vi "Write_Output.vi"(8 "Error_In":errorcluster, 10 "Output":dbl, 11 "Calculator_In":refnum<class "Calculator.lvclass">) -> (0 "Error_Out":errorcluster, 3 "Calculator_Out":refnum<class "Calculator.lvclass">)   [LabVIEW 2023, in "Calculator.lvclass"]
doc: "Used to write the data of output of calculator class"
uses:
  Calculator.lvclass
  Calculator.lvclass/Calculator.ctl
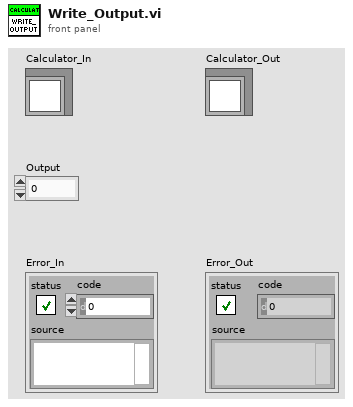
[diagram p1: front panel]
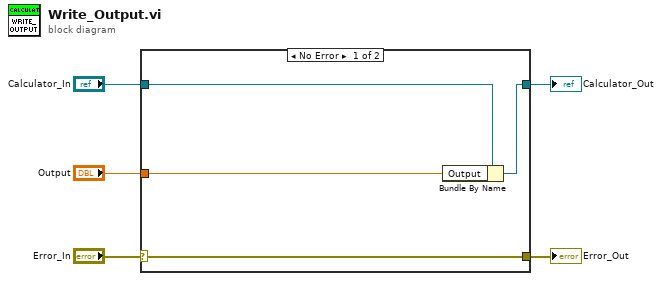
[diagram p0: block diagram]
diagram:
  n1 = case shown="No Error" "Error_In" {
    selector: "Error_In" -> [w9 w10]
    tunnel: [w9 w10] -> w4
    tunnel: [w7 w11] -> w2
    tunnel: "Calculator_In" -> [w8 w11]
    tunnel: "Output" -> [w6 _]
    frame No Error {
      n2 = Bundle By Name(cluster=w8, "Output"=w6) -> (w7:refnum<class "Calculator.lvclass">)
    }
    frame Error {
    }
  }
  "Error_Out" <- w4
  "Calculator_Out" <- w2
